vi "Sending Modulated Audio with SystemLink.vi"() -> ()   [LabVIEW 2019]
doc: "This application reads the selected audio file from its media storage. The audio is outputted through the EMONA Communications Board for its modulation. After being modulated, the signal is inputted once again into the application. The modulated signal is now displayed through the Modulated Signal Graph and also it is being sent to the other target by communicating with a TCP protocol.\nMeanwhile, the application also reads values from controls found at the Dashboard. This makes the process of communication much faster, as the two targets connect automatically by taking some configuration values from SystemLink Cloud."
uses:
  <vilib>/Skyline/Tag/Shared/typedefs/DataType.ctl
  <vilib>/myRIO/Instrument Drivers/Onboard IO/AI Continuous/typedefs/AI Continuous Reference.ctl
  <vilib>/myRIO/Common/Instrument Driver Framework/Utilities/typedefs/myRIO Generic Hardware Reference.ctl
  <vilib>/myRIO/Common/Instrument Driver Framework/Utilities/typedefs/Hardware Version Enum.ctl
  <vilib>/myRIO/Common/Instrument Driver Framework/Utilities/typedefs/myRIO v1.0 Reference.ctl
  <vilib>/myRIO/Common/Instrument Driver Framework/Utilities/typedefs/Generic FPGA Reference.ctl
  <vilib>/myRIO/Common/Instrument Driver Framework/ELVIS III v1.0/AI Continuous/typedefs/AI Continuous Channels List.ctl
  <vilib>/myRIO/Common/Instrument Driver Framework/ELVIS III v1.0/AI Continuous/typedefs/ELVIS III v1.0 AI Continuous Channels Enum.ctl
  <vilib>/myRIO/Common/Instrument Driver Framework/Utilities/typedefs/Analog Scaling Constants.ctl
  <vilib>/userDefined/High Color/nirio_resource_hc.ctl
  <vilib>/myRIO/Instrument Drivers/Onboard IO/AO Continuous/typedefs/AO Continuous Reference.ctl
  <vilib>/myRIO/Common/Instrument Driver Framework/ELVIS III v1.0/AO Continuous/typedefs/AO Continuous Channels List.ctl
  <vilib>/myRIO/Common/Instrument Driver Framework/ELVIS III v1.0/AO Continuous/typedefs/ELVIS III v1.0 AO Continuous Channels Enum.ctl
  <vilib>/myRIO/Common/Instrument Driver Framework/ELVIS III v1.0/AO Continuous/typedefs/AO Continuous Channel Info.ctl
  <vilib>/myRIO/Instrument Drivers/Onboard IO/AO/typedefs/AO Reference.ctl
  <vilib>/myRIO/Common/Instrument Driver Framework/myRIO v1.0/AO/typedefs/AO Channels List.ctl
  <vilib>/myRIO/Common/Instrument Driver Framework/myRIO v1.0/AO/typedefs/AO Channels Enum.ctl
  <vilib>/myRIO/Common/Instrument Driver Framework/Utilities/typedefs/Analog Scaling Constants List.ctl
  <vilib>/myRIO/Common/Instrument Driver Framework/ELVIS III v1.0/AI Continuous/vis/ELVIS III v1.1 Open AI (Continuous).vi
  <vilib>/myRIO/Common/Instrument Driver Framework/ELVIS III v1.0/AO Continuous/vis/ELVIS III v1.1 Open AO (Continuous).vi
  <vilib>/myRIO/Common/Instrument Driver Framework/ELVIS III v1.0/AO/vis/ELVIS III v1.1 Open AO.vi
  <vilib>/myRIO/Common/Instrument Driver Framework/Utilities/vis/Validate Channels.vi
  <vilib>/myRIO/Common/Instrument Driver Framework/ELVIS III v1.0/AI Continuous/vis/ELVIS III v1.0 Reserve AI Continuous.vi
  <vilib>/myRIO/Common/Instrument Driver Framework/ELVIS III v1.0/AO Continuous/vis/ELVIS III v1.0 Reserve AO Continuous.vi
  <vilib>/myRIO/Common/Instrument Driver Framework/ELVIS III v1.0/AO/vis/ELVIS III v1.0 Reserve AO.vi
  <vilib>/myRIO/Common/Instrument Driver Framework/ELVIS III v1.0/AO Continuous/vis/ELVIS III v1.1 Close AO Continuous.vi
  <vilib>/myRIO/Common/Instrument Driver Framework/ELVIS III v1.0/AO/vis/ELVIS III v1.0 Close AO.vi
  <vilib>/myRIO/Common/Instrument Driver Framework/ELVIS III v1.0/AI Continuous/vis/ELVIS III v1.0 Close AI Continuous.vi
  <vilib>/myRIO/Common/Instrument Driver Framework/myRIO v1.0/UART/vis/myRIO v1.0 Close UART.vi
  <vilib>/myRIO/Common/Instrument Driver Framework/ELVIS III v1.0/AI Continuous/vis/ELVIS III v1.0 Build MUX Configuration AI Continuous.vi
  <vilib>/myRIO/Common/Instrument Driver Framework/ELVIS III v1.0/AO Continuous/vis/ELVIS III v1.0 Build MUX Configuration AO Continuous.vi
  <vilib>/myRIO/Common/Instrument Driver Framework/ELVIS III v1.0/AO/vis/ELVIS III v1.0 Build MUX Configuration AO.vi
  <vilib>/myRIO/Common/Instrument Driver Framework/ELVIS III v1.0/AO Continuous/vis/ELVIS III v1.0 Unreserve AO Continuous.vi
  <vilib>/myRIO/Common/Instrument Driver Framework/ELVIS III v1.0/AO/vis/ELVIS III v1.0 Unreserve AO.vi
  <vilib>/myRIO/Common/Instrument Driver Framework/ELVIS III v1.0/AI Continuous/vis/ELVIS III v1.0 Unreserve AI Continuous.vi
  <vilib>/Skyline/Configuration/Configuration HTTP_class/Open Configuration API Key.vi
  <vilib>/Skyline/Tag/Wrapper/Wrapper HTTP_class/Open Tag HTTP.vi
  <vilib>/Skyline/Tag/Wrapper/Wrapper_class/Write Tag (Boolean).vi
  <vilib>/Skyline/Tag/Wrapper/Wrapper_class/Read Tag (String).vi
  <vilib>/Skyline/Tag/Wrapper/Wrapper_class/Close Tag (Single).vi
  <vilib>/Skyline/Tag/Wrapper/Wrapper_class/Read Tag (U64).vi
  <vilib>/Utility/VariantDataType/GetNumericInfo.vi
  <vilib>/Utility/error.llb/Error Cluster From Error Code.vi
  <vilib>/myRIO/Common/Instrument Driver Framework/ELVIS III v1.0/ELVIS III v1.1 Open.vi
  <vilib>/myRIO/Common/Instrument Driver Framework/ELVIS III v1.0/Resource Manager/vis/ELVIS III v1.0 Reserve Channel List.vi
  <vilib>/myRIO/Common/Instrument Driver Framework/myRIO v1.0/myRIO v1.0 Close.vi
  <vilib>/myRIO/Common/Instrument Driver Framework/ELVIS III v1.0/Resource Manager/vis/ELVIS III v1.0 Configure DMAs.vi
  <vilib>/myRIO/Common/Instrument Driver Framework/ELVIS III v1.0/AO Continuous/vis/ELVIS III v1.1 Stop AO Continuous.vi
  <vilib>/myRIO/Common/Instrument Driver Framework/ELVIS III v1.0/Resource Manager/vis/ELVIS III v1.0 Coerce AI Scaling.vi
  <vilib>/myRIO/Common/Instrument Driver Framework/ELVIS III v1.0/AI Continuous/vis/ELVIS III v1.1 Stop AI Continuous.vi
  <vilib>/myRIO/Common/Instrument Driver Framework/ELVIS III v1.0/AI Continuous/vis/ELVIS III v1.1 Start AI Continuous.vi
  <vilib>/Skyline/Tag/Wrapper/Wrapper_class/Read Tag (Boolean).vi
  <vilib>/myRIO/Common/Instrument Driver Framework/ELVIS III v1.0/AO Continuous/vis/ELVIS III v1.0 AO Continuous Write.vi
  <vilib>/myRIO/Common/Instrument Driver Framework/ELVIS III v1.0/AO/vis/ELVIS III v1.0 Write AO.vi
  <vilib>/myRIO/Common/Instrument Driver Framework/ELVIS III v1.0/AO Continuous/vis/ELVIS III v1.1 Start AO Continuous.vi
  <vilib>/myRIO/Common/Instrument Driver Framework/ELVIS III v1.0/AI Continuous/vis/ELVIS III v1.0 AI Continuous Read.vi
  <vilib>/myRIO/Common/Instrument Driver Framework/ELVIS III v1.0/Resource Manager/vis/ELVIS III v1.0 Unreserve Channel List.vi
  <vilib>/myRIO/Common/Instrument Driver Framework/Utilities/vis/FPGA Ref Manager.vi
  <vilib>/myRIO/Common/Instrument Driver Framework/ELVIS III v1.0/ELVIS III v1.0 Reset FPGA.vi
  <vilib>/myRIO/Common/Instrument Driver Framework/myRIO v1.0/IRQ/vis/myRIO v1.0 IRQ Info FGV.vi
  <vilib>/myRIO/Common/Instrument Driver Framework/myRIO v1.0/IRQ/vis/myRIO v1.0 Timer IRQ Info FGV.vi
  <vilib>/myRIO/Common/Instrument Driver Framework/myRIO v1.0/IRQ/vis/myRIO v1.0 ISR Agent.vi
  <vilib>/myRIO/Instrument Drivers/Utilities/vis/Reset Index.vi
  <vilib>/myRIO/Common/Instrument Driver Framework/myRIO v1.0/Resource Manager/vis/myRIO v1.0 Block Write Resource Manager.vi
  <vilib>/myRIO/Instrument Drivers/Onboard IO/AO/vis/myRIO AO Open.xnode
  <vilib>/myRIO/Instrument Drivers/Onboard IO/AO Continuous/vis/myRIO AO Continuous Open.xnode
  <vilib>/myRIO/Instrument Drivers/Onboard IO/AI Continuous/vis/myRIO AI Continuous Open.xnode
  <vilib>/myRIO/Instrument Drivers/Utilities/Utilities.lvlib
  <vilib>/myRIO/Instrument Drivers/Onboard IO/AO/AO.lvlib
  <vilib>/myRIO/Instrument Drivers/Onboard IO/AO Continuous/AO Continuous.lvlib
  <vilib>/myRIO/Instrument Drivers/Onboard IO/AI Continuous/AI Continuous.lvlib
  <vilib>/Skyline/Configuration/Configuration_class/NI Skyline Configuration.lvclass
  <vilib>/Skyline/Tag/Wrapper/Wrapper_class/NI Skyline Tag.lvclass
  <vilib>/Skyline/Tag/Shared/NI Skyline Tag.lvlib
  <vilib>/Skyline/Tag/Wrapper/Wrapper HTTP_class/NI Skyline Tag HTTP.lvclass
  <vilib>/Skyline/Configuration/Configuration HTTP_class/NI Skyline Configuration HTTP.lvclass
panel:
  in  "Stop":bool
  out "Select Audio":u16(ring) items=["ABBA- Dancing Queen.mp3", "Frank Sinatra - Fly Me To The Moon.mp3", "Gotye - Somebody That I Used To Know.mp3", "Mozart - Eine Kleine Nachtmusik.mp3"]
  in  "Address":string caption="Demodulator IP Address"
  out "Message":dbl[](graph) caption="Message History"
  in  "Offset":dbl=2.0
  out "Modulated Signal":dbl[](graph)
  out "error out":errorcluster
  # "Sending and Modulating Audio"
  # "Explanation:\nThis application reads the selected audio file from its media storage. The audio is outputted through the EMONA Communications Board for its modulation. After being modulated, the signal is inputted once again into the application. The modulated signal is now displayed through the Modulated Signal Graph and also it is being sent to the other target by communicating with a TCP protocol.\nMeanwhile, the application also reads values from controls found at the Dashboard. This makes the process of communication much faster, as the two targets connect automatically by taking some configuration values from SystemLink Cloud.\n \nInstructions:\nOpen the Audio Modulation Dashboard shortcut from the project folder. There you will find the controls to change the values from the VIs. Also shutdown the application through the Stop switch at the Dashboard. Remember to always run the Receiving Modulated Audio VI before running this one. Check the instructions on the other VI for more information."
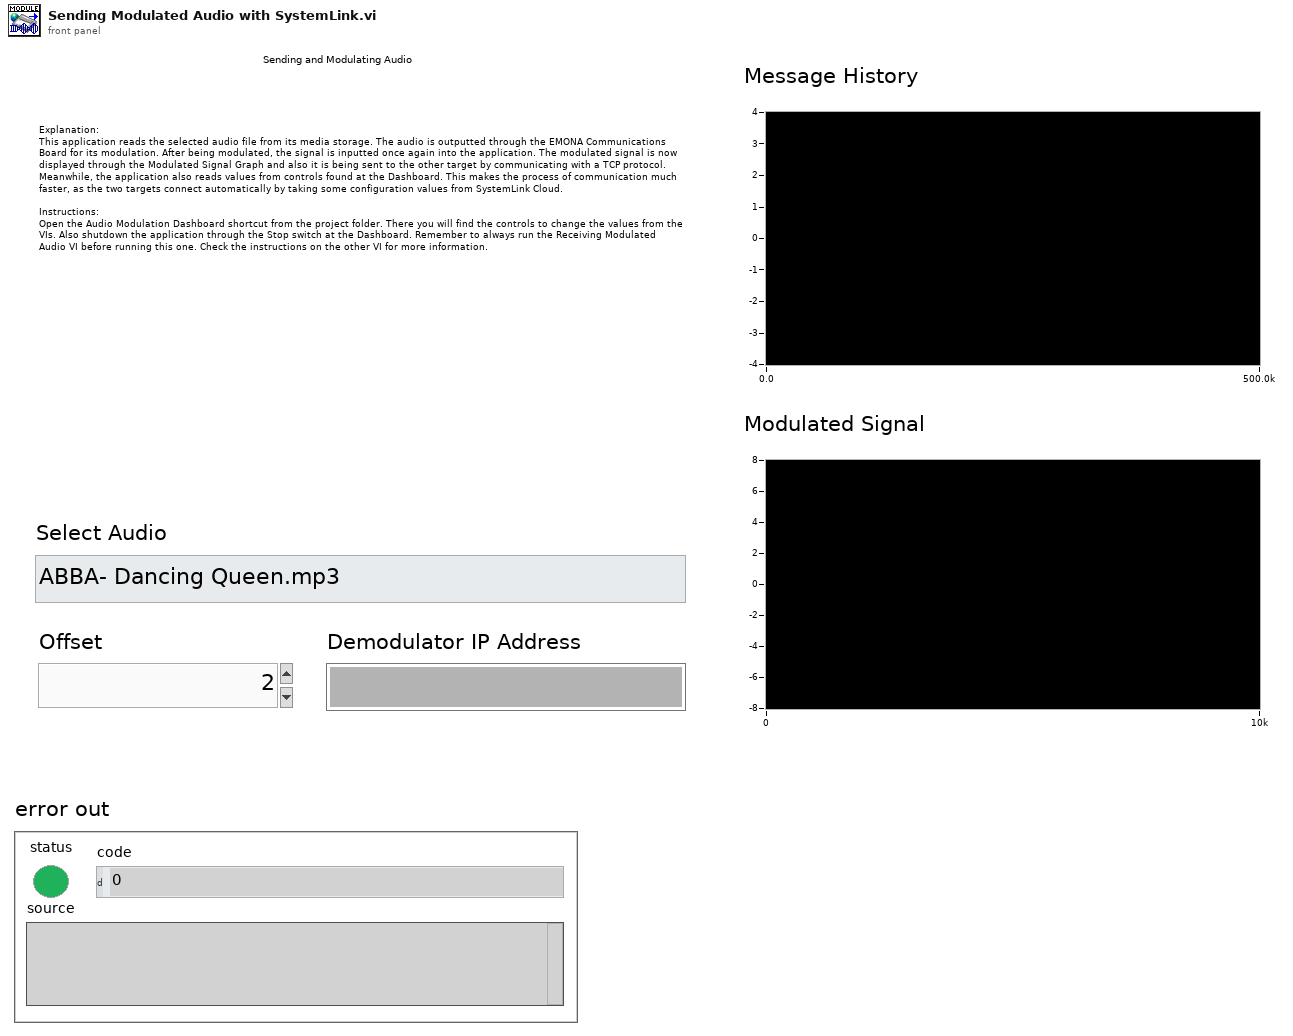
[diagram p1: front panel]
types:
  T1 = typedef "NI Skyline Tag.lvlib/DataType.ctl" = enum32{"Double", "I32", "String", "Boolean", "U64", "Timestamp"}
  T2 = enum16{"open", "replace", "create", "open or create", "replace or create", "replace or create with confirmation"}
  T3 = typedef "AI Continuous.lvlib/AI Continuous Reference.ctl" = cluster{"myRIO Reference":T4, "AI (Continuous) Channels List":T8, "AI (Continuous) Scaling Constants List":T10[], "Bank Count":u8[]}
  T4 = typedef "myRIO Generic Hardware Reference.ctl" = cluster{"myRIO Model":T5, "myRIO Hardware Reference":T6}
  T5 = typedef "Hardware Version Enum.ctl" = enum16{"Unknown", "myRIO-1900", "myRIO-1950", "roboRIO", "NI ELVIS RIO CM", "ELVIS III"}
  T6 = typedef "myRIO v1.0 Reference.ctl" = cluster{"Generic FPGA Reference":T7, "Allow multiple opens":bool}
  T7 = typedef "Generic FPGA Reference.ctl" = refnum<k20>
  T8 = typedef "AI Continuous Channels List.ctl" = T9[]
  T9 = typedef "ELVIS III v1.0 AI Continuous Channels Enum.ctl" = enum16{"Not Connected", "A/AI0 (Continuous)", "A/AI1 (Continuous)", "A/AI2 (Continuous)", "A/AI3 (Continuous)", "A/AI4 (Continuous)", "A/AI5 (Continuous)", "A/AI6 (Continuous)", "A/AI7 (Continuous)", "A/AI0 (DIFF Continuous)", "A/AI1 (DIFF Continuous)", "A/AI2 (DIFF Continuous)", "A/AI3 (DIFF Continuous)", "B/AI0 (Continuous)", "B/AI1 (Continuous)", "B/AI2 (Continuous)", "B/AI3 (Continuous)", "B/AI4 (Continuous)", "B/AI5 (Continuous)", "B/AI6 (Continuous)", "B/AI7 (Continuous)", "B/AI0 (DIFF Continuous)", "B/AI1 (DIFF Continuous)", "B/AI2 (DIFF Continuous)", "B/AI3 (DIFF Continuous)"}
  T10 = typedef "Analog Scaling Constants.ctl" = cluster{"LSB Weight (Volts)":dbl, "Offset (Volts)":dbl, "Signed?":bool}
  T11 = typedef "AO Continuous.lvlib/AO Continuous Reference.ctl" = cluster{"myRIO Reference":T4, "AO (Continuous) Channels List":T12, "Channel Info":T14}
  T12 = typedef "AO Continuous Channels List.ctl" = T13[]
  T13 = typedef "ELVIS III v1.0 AO Continuous Channels Enum.ctl" = enum16{"Not Connected", "A/AO0 (Continuous)", "A/AO1 (Continuous)", "B/AO0 (Continuous)", "B/AO1 (Continuous)"}
  T14 = typedef "AO Continuous Channel Info.ctl" = cluster{"Channel Bitmask":u8[], "Channel Index":i32[], "Channel Number":u8}
  T15 = typedef "AO.lvlib/AO Reference.ctl" = cluster{"myRIO Reference":T4, "AO Channel List":T16, "AO Scaling Constant List":T18}
  T16 = typedef "AO Channels List.ctl" = T17[]
  T17 = typedef "AO Channels Enum.ctl" = enum16{"Not Connected", "AudioOut/Left", "AudioOut/Right", "C/AO0", "C/AO1", "A/AO0", "A/AO1", "B/AO0", "B/AO1"}
  T18 = typedef "Analog Scaling Constants List.ctl" = T10[]
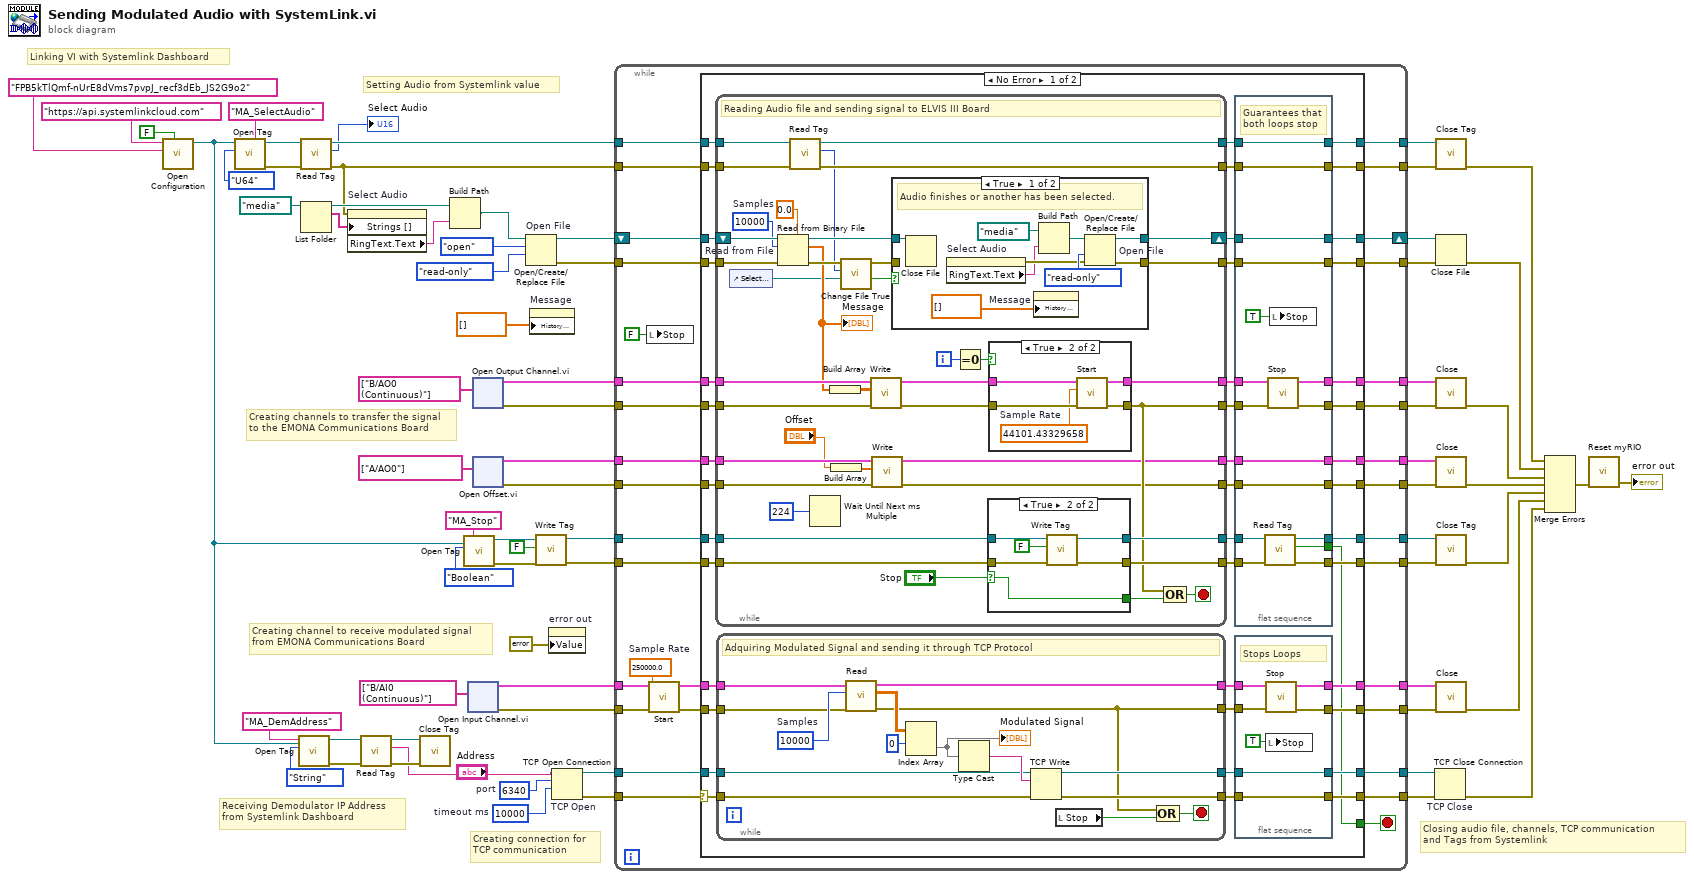
[diagram p0: block diagram]
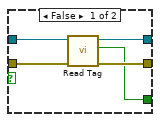
[diagram p3: hidden frame]
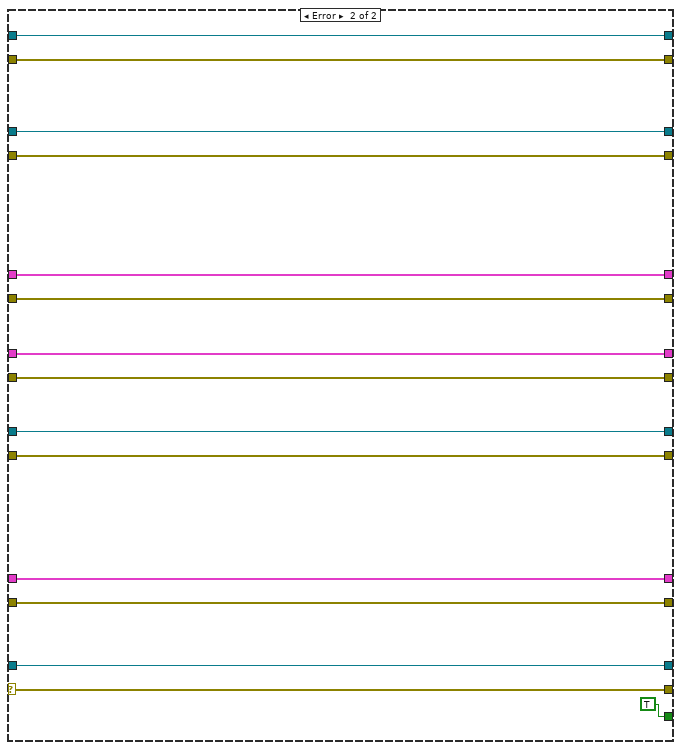
[diagram p5: hidden frame]
diagram:
  w20 = 10000  # timeout ms
  w19 = u16 6340  # port
  # "Closing audio file, channels, TCP communication\nand Tags from Systemlink"
  # "Setting Audio from Systemlink value"
  # "Creating connection for\nTCP communication"
  # "Receiving Demodulator IP Address\nfrom Systemlink Dashboard"
  # "Creating channel to receive modulated signal\nfrom EMONA Communications Board"
  # "Creating channels to transfer the signal\nto the EMONA Communications Board"
  # "Linking VI with Systemlink Dashboard"
  n1 = call-poly <vilib>:"Open Configuration.vi"("verify server?"=FALSE, "api key"="FPB5kTlQmf-nUrE8dVms7pvpJ_recf3dEb_JS2G9o2", "server url"="https://api.systemlinkcloud.com") -> ("HTTP configuration out"=w11:refnum<class "NI Skyline Configuration HTTP.lvclass">)  [unwired: 7 in, 1 out]
  n2 = call-poly <vilib>:"Open Tag.vi"("configuration"=w11, "Data Type"=DataType."U64", "path"="MA_SelectAudio") -> ("error out"=w27:errorcluster, "tag out"=w28:refnum<class "NI Skyline Tag.lvclass">)  [unwired: 7 in]
  n3 = call-poly <vilib>:"Open Tag.vi"("configuration"=w11, "Data Type"=DataType."String", "path"="MA_DemAddress") -> ("error out"=w36:errorcluster, "tag out"=w37:refnum<class "NI Skyline Tag.lvclass">)  [unwired: 7 in]
  n4 = call-poly <vilib>:"Read Tag.vi"("error in (no error)"=w27, "tag in"=w28) -> ("error out"=w4:errorcluster, "value"=→"Select Audio":u64, "tag out"=w6:refnum<class "NI Skyline Tag.lvclass">)  [unwired: 5 in, 2 out]
  n5 = List Folder(path=path "/media") -> (path out=w32:path, filenames=w3:string[])  [unwired: 3 in, 2 out]
  n6 = property on="Select Audio" class="Ring (strict)"(error in=w4, "Strings []"=w3) -> ("RingText.Text"=w2:string)  [unwired: 1 in, 2 out]
  n7 = call-poly <vilib>:"Read Tag.vi"("error in (no error)"=w36, "tag in"=w37) -> ("error out"=w34:errorcluster, "value"=w16:string, "tag out"=w35:refnum<class "NI Skyline Tag.lvclass">)  [unwired: 5 in, 2 out]
  n8 = call-poly <vilib>:"Close Tag.vi"("error in (no error)"=w34, "tag in"=w35) -> ()  [unwired: 9 in, 1 out]
  n9 = Build Path(base path=w32, name or relative path=w2) -> (appended path=w31:path)
  n10 = call-poly <vilib>:"Open Tag.vi"("configuration"=w11, "Data Type"=DataType."Boolean", "path"="MA_Stop") -> ("error out"=w41:errorcluster, "tag out"=w42:refnum<class "NI Skyline Tag.lvclass">)  [unwired: 7 in]
  n11 = xnode "Open Input Channel.vi"("Channel Names"=tag[] ["B/AI0 (Continuous)"]) -> ("error out"=w17:errorcluster, "AI (Continuous) Ref Out"=w59:T3)  [unwired: 3 in]
  n12 = xnode "Open Output Channel.vi"("Channel Names"=tag[] ["B/AO0 (Continuous)"]) -> ("error out"=w66:errorcluster, "AO (Continuous) Ref Out"=w67:T11)  [unwired: 1 in]
  n13 = xnode "Open Offset.vi"("Channel Names"=tag[] ["A/AO0"]) -> ("error out"=w71:errorcluster, "AO Ref Out"=w72:T15)  [unwired: 2 in]
  n14 = Open/Create/Replace File "Open File"(file path (use dialog)=w31, operation (0:open)=T2."open", access (0:read/write)=enum16{"read/write", "read-only", "write-only"}."read-only") -> (refnum out=w69:refnum<file>, error out=w68:errorcluster)  [unwired: 3 in, 1 out]
  n15 = property on="Message" class="WFChart (strict)"("History Data"=dbl[] []) -> ()  [unwired: 2 in, 2 out]
  n16 = call-poly <vilib>:"Write Tag.vi"("error in (no error)"=w41, "value"=FALSE, "tag in"=w42) -> ("error out"=w57:errorcluster, "tag out"=w58:refnum<class "NI Skyline Tag.lvclass">)  [unwired: 7 in]
  n17 = property on="error out" class="Clust (strict)"("Value"=errorcluster {"status"=FALSE, "code"=0, "source"=""} ("error constant")) -> ()  [unwired: 2 in, 2 out]
  n18 = TCP Open Connection "TCP Open"(address=w16, remote port or service name=w19, timeout ms (60000)=w20) -> (connection ID=w18:refnum<k5>, error out=w14:errorcluster)  [unwired: 2 in]
  n19 = while {
    shift-right: [w96] -> w63
    shift-left: w69 -> [w102]
    tunnel: w59 -> [w92]
    tunnel: [w95] -> w62
    tunnel: w57 -> [w90]
    tunnel: [w88] -> w55
    tunnel: w58 -> [w91]
    tunnel: [w89] -> w56
    tunnel: w71 -> [w104]
    tunnel: [w103] -> w70
    tunnel: w72 -> [w105]
    tunnel: [w98] -> w65
    tunnel: w67 -> [w100]
    tunnel: [w93] -> w60
    tunnel: w66 -> [w99]
    tunnel: [w94] -> w61
    tunnel: w68 -> [w101]
    tunnel: [w97] -> w64
    tunnel: w4 -> [w87]
    tunnel: [w85] -> w54
    tunnel: w6 -> [w86]
    tunnel: [w84] -> w53
    tunnel: [w79] -> w23
    tunnel: [w78] -> w21
    tunnel: w18 -> [w77]
    tunnel: w17 -> [w76]
    tunnel: w14 -> [w74]
    tunnel: [w75] -> w13
    stop <- w73 stop-if-true
    w83 = 250000.0  # Sample Rate
    n20 = local write "Stop"(FALSE ("Stop")) -> ()
    n21 = call <vilib>:"Start.vi"("error in (no error)"=w76, "Sample Rate"=w83, "AI (Continuous) Ref In"=w92) -> ("error out"=w81:errorcluster, "AI (Continuous) Ref Out"=w82:T3)  [unwired: 7 in]
    n22 = case shown="No Error" w74 {
      selector: w74 -> [w107 w257]
      tunnel: w105 -> [w148 w264]
      tunnel: w104 -> [w147 w263]
      tunnel: [w146 w263] -> w103
      tunnel: w102 -> [w145 w268]
      tunnel: w101 -> [w144 w267]
      tunnel: w100 -> [w143 w266]
      tunnel: w99 -> [w142 w265]
      tunnel: [w141 w264] -> w98
      tunnel: [w140 w267] -> w97
      tunnel: [w139 w268] -> w96
      tunnel: [w138 w260] -> w95
      tunnel: [w137 w265] -> w94
      tunnel: [w136 w266] -> w93
      tunnel: w91 -> [w135 w262]
      tunnel: w90 -> [w134 w261]
      tunnel: [w133 w262] -> w89
      tunnel: [w132 w261] -> w88
      tunnel: w87 -> [w131 w269]
      tunnel: w86 -> [w130 w270]
      tunnel: [w129 w269] -> w85
      tunnel: [w128 w270] -> w84
      tunnel: w82 -> [w118 w260]
      tunnel: w81 -> [w113 w259]
      tunnel: [w112 w259] -> w79
      tunnel: [w111 w258] -> w78
      tunnel: w77 -> [w110 w258]
      tunnel: [w108 w257] -> w75
      tunnel: [w106 TRUE ("value")] -> w73
      frame No Error {
        n23 = while {
          tunnel: w148 -> [w195]
          tunnel: w147 -> [w196]
          tunnel: [w194] -> w126
          tunnel: [w193] -> w127
          tunnel: w144 -> [w224]
          tunnel: [w208] -> w123
          tunnel: w142 -> [w216]
          tunnel: [w197] -> w125
          tunnel: w143 -> [w217]
          tunnel: [w215] -> w124
          tunnel: w135 -> [w212]
          tunnel: w134 -> [w213]
          tunnel: [w211] -> w117
          tunnel: [w204] -> w116
          shift-right: [w209] -> w122
          shift-left: w145 -> [w225]
          tunnel: w131 -> [w203]
          tunnel: w130 -> [w202]
          tunnel: [w201] -> w115
          tunnel: [w200] -> w114
          i -> [w218]
          stop <- w226 stop-if-true
          w222 = 10000  # Samples
          # "Reading Audio file and sending signal to ELVIS III Board"
          n24 = control-ref of="Select Audio"() -> (w187:refnum<vi>)
          n25 = Read from Binary File "Read from File"(5:0.0, 8:w224, 10:w222, 11:w225) -> (0:w207:errorcluster, 2:w188:dbl[], 3:w210:refnum<file>)  [unwired: 2 in, 1 out]
          "Message" <- w188
          n26 = call-poly <vilib>:"Read Tag.vi"("error in (no error)"=w203, "tag in"=w202) -> ("error out"=w201:errorcluster, "value"=w199:u64, "tag out"=w200:refnum<class "NI Skyline Tag.lvclass">)  [unwired: 5 in, 2 out]
          n27 = Wait Until Next ms Multiple(millisecond multiple=u32 224) -> ()  [unwired: 1 out]
          n28 = Build Array(w188) -> (w214:dbl[][])
          n29 = Build Array("Offset") -> (w192:dbl[])
          n30 = call "Change File True.vi"("error in"=w207, "Numeric in"=w199, "Ring"=w187) -> ("error out"=w206:errorcluster, "Change song?"=w205:bool)  [unwired: 5 in, 1 out]
          n31 = call <vilib>:"Write.vi"("error in (no error)"=w216, "Data To Write"=w214, "AO (Continuous) Ref In"=w217) -> ("error out"=w220:errorcluster, "AO (Continuous) Ref Out"=w221:T11)  [unwired: 7 in]
          n32 = call <vilib>:"Write.vi"("error in (no error)"=w196, "Values"=w192, "AO Ref In"=w195) -> ("error out"=w193:errorcluster, "AO Ref Out"=w194:T15)  [unwired: 6 in]
          n33 = case shown="True" w205 {
            tunnel: [w233 w236] -> w208
            tunnel: w210 -> [w235 w237]
            tunnel: [w234 w237] -> w209
            tunnel: w206 -> [_ w236]
            frame True {
              # "Audio finishes or another has been selected."
              n34 = Close File(refnum=w235) -> ()  [unwired: 1 in, 2 out]
              n35 = property on="Select Audio" class="Ring (strict)"() -> (error out=w228:errorcluster, "RingText.Text"=w227:string)  [unwired: 2 in, 1 out]
              n36 = property on="Message" class="WFChart (strict)"("History Data"=dbl[] []) -> ()  [unwired: 2 in, 2 out]
              n37 = Build Path(base path=path "/media" ("path"), name or relative path=w227) -> (appended path=w231:path)
              n38 = Open/Create/Replace File "Open File"(file path (use dialog)=w231, error in=w228, access (0:read/write)=enum16{"read/write", "read-only", "write-only"}."read-only") -> (refnum out=w234:refnum<file>, error out=w233:errorcluster)  [unwired: 3 in, 1 out]
            }
            frame False {
              # "Nothing occured"
            }
          }
          n39 = Equal To 0?(x=w218) -> (x = 0?=w219:bool)
          n40 = case shown="True" "Stop" {
            selector: "Stop" -> [_ w246]
            tunnel: w213 -> [w241 w248]
            tunnel: w212 -> [w242 w247]
            tunnel: [w238 w246] -> w198
            tunnel: [w240 w245] -> w211
            tunnel: [w239 w244] -> w204
            frame False {
              n41 = call-poly <vilib>:"Read Tag.vi"("error in (no error)"=w241, "tag in"=w242) -> ("error out"=w239:errorcluster, "value"=w238:bool, "tag out"=w240:refnum<class "NI Skyline Tag.lvclass">)  [unwired: 5 in, 2 out]
            }
            frame True {
              n42 = call-poly <vilib>:"Write Tag.vi"("error in (no error)"=w248, "value"=FALSE, "tag in"=w247) -> ("error out"=w244:errorcluster, "tag out"=w245:refnum<class "NI Skyline Tag.lvclass">)  [unwired: 7 in]
            }
          }
          n43 = case shown="True" w219 {
            tunnel: w221 -> [w250 w255]
            tunnel: w220 -> [w249 w254]
            tunnel: [w250 w253] -> w215
            tunnel: [w249 w252] -> w197
            frame False {
            }
            frame True {
              w251 = 44101.43329658  # Sample Rate
              n44 = call <vilib>:"Start.vi"("error in (no error)"=w254, "Sample Rate"=w251, "AO (Continuous) Ref In"=w255) -> ("error out"=w252:errorcluster, "AO (Continuous) Ref Out"=w253:T11)  [unwired: 7 in]
            }
          }
          n45 = Compound Arithmetic op=OR(w197, w198) -> (w226:bool)
        }
        n46 = while {
          tunnel: [w181] -> w121
          tunnel: [w173] -> w120
          tunnel: w110 -> [w178]
          tunnel: [w179] -> w119
          tunnel: w118 -> [w177]
          tunnel: w113 -> [w176]
          tunnel: w107 -> [w175]
          tunnel: [w174] -> w109
          stop <- w185 stop-if-true
          w183 = u32 10000  # Samples
          # "Adquiring Modulated Signal and sending it through TCP Protocol"
          n47 = call <vilib>:"Read.vi"("error in (no error)"=w176, "Number of Samples"=w183, "AI (Continuous) Ref In"=w177) -> ("error out"=w173:errorcluster, "Values"=w182:dbl[][], "AI (Continuous) Ref Out"=w181:T3)  [unwired: 6 in]
          n48 = Index Array(array=w182, index (row)=0) -> (element=w172:dbl[])  [unwired: 1 in]
          "Modulated Signal" <- w172
          n49 = Type Cast(x=w172) -> (*(type *) &x=w180:string)  [unwired: 1 out]
          n50 = TCP Write(connection ID=w178, data in=w180, error in (no error)=w175) -> (connection ID out=w179:refnum<k5>, error out=w174:errorcluster)  [unwired: 2 out]
          n51 = local read "Stop"() -> (w184:bool)
          n52 = Compound Arithmetic op=OR(w173, w184) -> (w185:bool)
        }
        n53 = flat-sequence {
          tunnel: w127 -> [w171]
          tunnel: [w171] -> w146
          tunnel: [w170] -> w141
          tunnel: w126 -> [w170]
          tunnel: w125 -> [w163]
          tunnel: w124 -> [w164]
          tunnel: [w169] -> w140
          tunnel: w123 -> [w169]
          tunnel: w122 -> [w168]
          tunnel: [w168] -> w139
          tunnel: [w166] -> w137
          tunnel: [w165] -> w136
          tunnel: w117 -> [w159]
          tunnel: w116 -> [w158]
          tunnel: [w160] -> w133
          tunnel: [w157] -> w132
          tunnel: [w162] -> w129
          tunnel: w115 -> [w162]
          tunnel: w114 -> [w161]
          tunnel: [w161] -> w128
          tunnel: [w156] -> w106
          frame #0 {
            # "Guarantees that both loops stop"
            n54 = call-poly <vilib>:"Read Tag.vi"("error in (no error)"=w158, "tag in"=w159) -> ("error out"=w157:errorcluster, "value"=w156:bool, "tag out"=w160:refnum<class "NI Skyline Tag.lvclass">)  [unwired: 5 in, 2 out]
            n55 = call <vilib>:"Stop.vi"("error in (no error)"=w163, "AO (Continuous) Ref In"=w164) -> ("error out"=w166:errorcluster, "AO (Continuous) Ref Out"=w165:T11)  [unwired: 8 in]
            n56 = local write "Stop"(TRUE ("Stop")) -> ()
          }
        }
        n57 = flat-sequence {
          tunnel: w121 -> [w153]
          tunnel: w120 -> [w152]
          tunnel: [w154] -> w138
          tunnel: w119 -> [w150]
          tunnel: [w151] -> w112
          tunnel: [w150] -> w111
          tunnel: w109 -> [w149]
          tunnel: [w149] -> w108
          frame #0 {
            # "Stops Loops"
            n58 = call <vilib>:"Stop.vi"("error in (no error)"=w152, "AI (Continuous) Ref In"=w153) -> ("error out"=w151:errorcluster, "AI (Continuous) Ref Out"=w154:T3)  [unwired: 8 in]
            n59 = local write "Stop"(TRUE ("Stop")) -> ()
          }
        }
      }
      frame Error {
      }
    }
  }
  n60 = TCP Close Connection "TCP Close"(connection ID=w21, error in (no error)=w13) -> (error out=w12:errorcluster)  [unwired: 2 out]
  n61 = call-poly <vilib>:"Close Tag.vi"("error in (no error)"=w54, "tag in"=w53) -> ("error out"=w8:errorcluster)  [unwired: 9 in]
  n62 = Close File(refnum=w63, error in=w64) -> (error out=w9:errorcluster)  [unwired: 1 out]
  n63 = call <vilib>:"Close.vi"("error in (no error)"=w61, "AO (Continuous) Ref In"=w60) -> ("error out"=w10:errorcluster)  [unwired: 9 in]
  n64 = call <vilib>:"Close.vi"("error in (no error)"=w70, "AO Ref In"=w65) -> ("error out"=w25:errorcluster)  [unwired: 9 in]
  n65 = call-poly <vilib>:"Close Tag.vi"("error in (no error)"=w55, "tag in"=w56) -> ("error out"=w24:errorcluster)  [unwired: 9 in]
  n66 = call <vilib>:"Close.vi"("error in (no error)"=w23, "AI (Continuous) Ref In"=w62) -> ("error out"=w22:errorcluster)  [unwired: 9 in]
  n67 = Merge Errors(w8, w9, w10, w25, w24, w22, w12) -> (w15:errorcluster)
  n68 = call <vilib>:"Reset myRIO.vi"("error in (no error)"=w15) -> ("error out"=→"error out":errorcluster)  [unwired: 10 in]
